vi "Commit NVMEM (Core).vi"(7 "nvmem type":T1, 8 "error in (no error)":errorcluster, 10 "resources":string, 11 "SLSC Remote in":refnum<class "SLSC Remote.lvclass">) -> (0 "error out":errorcluster, 3 "SLSC Remote out":refnum<class "SLSC Remote.lvclass">)   [LabVIEW 2015, in "SLSC Remote.lvclass"]
uses:
  SLSC Remote.lvclass
  SLSC Interface Class/nvmem type.ctl
  <vilib>/NI/i3 JSON/JSON Generation/Create Value Files/Create Value - Object.vi
  <vilib>/NI/i3 JSON/JSON Generation/Add Object Parameter Files/Add Object Parameter - String.vi
  <vilib>/NI/NI JSONRPC Server Framework/Classes/Server/Format Client Request (Auto-Increment).vi
  <vilib>/httpClient/POSTBuffer.vi
  <vilib>/NI/NI JSONRPC Server Framework/Classes/Server/JSONRPC Server.lvclass
  <vilib>/NI/i3 JSON/i3-json.lvlib
  <vilib>/httpClient/LabVIEWHTTPClient.lvlib
  SLSC Interface Class/SLSC Interface.lvclass
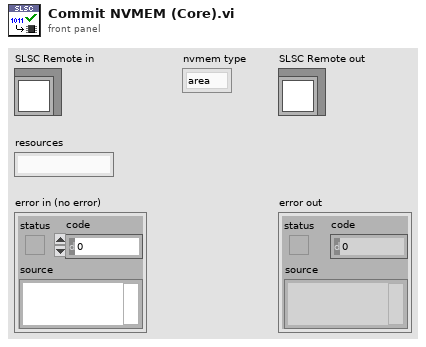
[diagram p1: front panel]
types:
  T1 = typedef "SLSC Interface.lvclass/nvmem type.ctl" = enum16{"area", "device", "session"}
  T2 = typedef "LabVIEWHTTPClient.lvlib/ClientHandle.ctl" = refnum<k1>
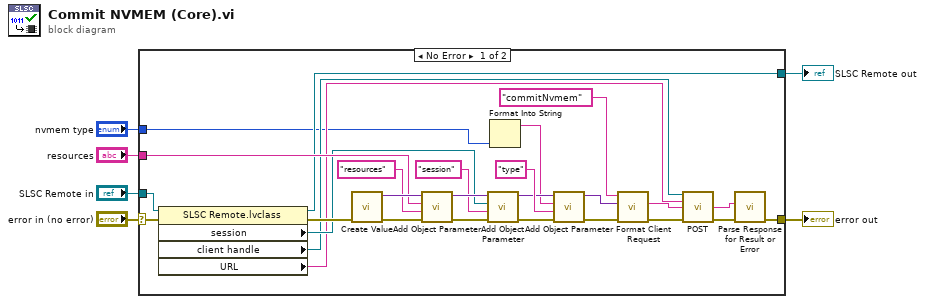
[diagram p0: block diagram]
diagram:
  n1 = case shown="No Error" "error in (no error)" {
    selector: "error in (no error)" -> [w28 w34]
    tunnel: "resources" -> [w32 _]
    tunnel: "SLSC Remote in" -> [w30 w35]
    tunnel: [w29 w35] -> w4
    tunnel: [w14 w34] -> w2
    tunnel: "nvmem type" -> [w8 _]
    frame No Error {
      n2 = property class="SLSC Remote.lvclass"(reference=w30, error in=w28) -> (reference out=w29:refnum<class "SLSC Remote.lvclass">, error out=w27:errorcluster, "session"=w21:refnum<k21>, "client handle"=w19:T2, "URL"=w18:string)
      n3 = call-poly <vilib>:"Create Value.vi"("error in (no error)"=w27) -> ("error out"=w26:errorcluster, "JSON Tree"=w33:variant)  [unwired: 9 in]
      n4 = call-poly <vilib>:"Add Object Parameter.vi"("error in (no error)"=w26, "Name"="resources", "String"=w32, "JSON Tree in (JSON Object)"=w33) -> ("error out"=w25:errorcluster, "JSON Tree out (JSON Object)"=w22:variant)  [unwired: 6 in]
      n5 = call-poly <vilib>:"Add Object Parameter.vi"("error in (no error)"=w25, "Name"="session", "String"=w21, "JSON Tree in (JSON Object)"=w22) -> ("error out"=w10:errorcluster, "JSON Tree out (JSON Object)"=w12:variant)  [unwired: 6 in]
      n6 = Format Into String(w8) -> (resulting string=w7:string)  [unwired: 3 in, 1 out]
      n7 = call-poly <vilib>:"Add Object Parameter.vi"("error in (no error)"=w10, "Name"="type", "String"=w7, "JSON Tree in (JSON Object)"=w12) -> ("error out"=w9:errorcluster, "JSON Tree out (JSON Object)"=w11:variant)  [unwired: 6 in]
      n8 = call-poly <vilib>:"Format Client Request.vi"("error in (no error)"=w9, "params"=w11, "method"="commitNvmem") -> ("error out"=w17:errorcluster, "Request String"=w23:string)  [unwired: 7 in]
      n9 = call-poly <vilib>:"POST.vi"("client handle"=w19, "url"=w18, "buffer"=w23, "error in (no error)"=w17) -> ("body"=w16:string, "error out"=w15:errorcluster)  [unwired: 8 in, 2 out]
      n10 = call <vilib>:"Parse Response for Result or Error.vi"("error in"=w15, "Response String In"=w16) -> ("error out"=w14:errorcluster)  [unwired: 7 in, 2 out]
    }
    frame Error {
    }
  }
  "error out" <- w2
  "SLSC Remote out" <- w4
